vi "From String Array.vi"(8 "error in (no error)":errorcluster, 9 "String Array":string[](array[string]), 11 "Parallel Step Config in":refnum<class "Parallel Step Config.lvclass">) -> (0 "error out":errorcluster, 1 "Elements Left":string[](array[string]), 3 "Parallel Step Config out":refnum<class "Parallel Step Config.lvclass">)   [LabVIEW 2015, in "Parallel Step Config.lvclass"]
uses:
  Parallel Step Config.lvclass
  classes/Step/Config/Step Config.lvclass
panel:
  out "Elements Left 2":string[][](array[string])
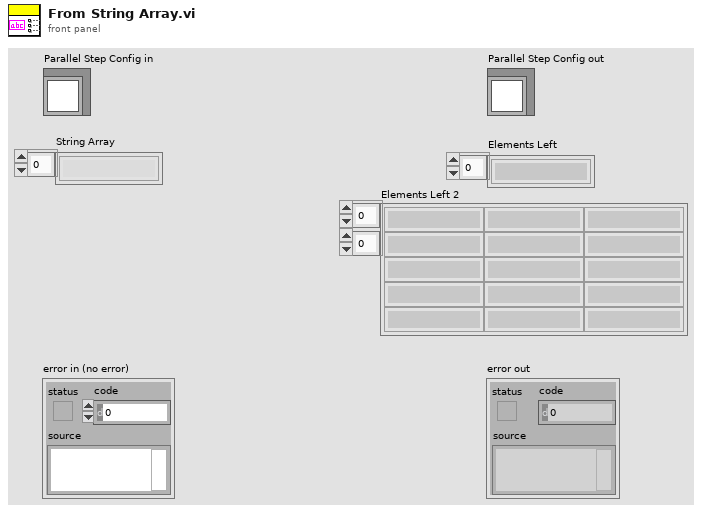
[diagram p1: front panel]
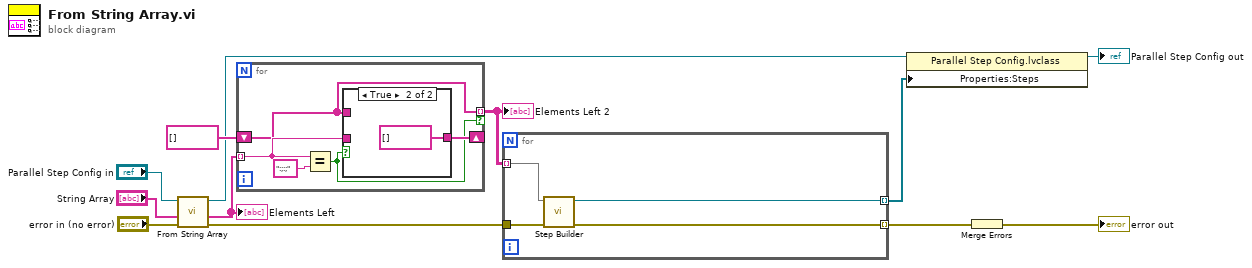
[diagram p0: block diagram]
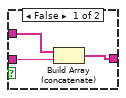
[diagram p2: hidden frame]
diagram:
  n1 = call-parent "From String Array.vi"("error in (no error)"="error in (no error)", "String Array"="String Array", "Step Config in"="Parallel Step Config in") -> ("error out"=w6:errorcluster, "Elements Left 2"=w9:string[], "Step Config out"=w3:refnum<class "Parallel Step Config.lvclass">)  [unwired: 6 in]
  "Elements Left" <- w9
  n2 = for {
    tunnel: w9 -> [w15] mode=indexing
    shift-right: [w16] -> _
    shift-left: string[] [] ("Elements Left 2") -> [w14]
    tunnel: [w14] -> w7 mode=indexing if=w13
    n3 = Equal?(x=w15, y=":;:;") -> (x = y?=w13:bool)
    n4 = case shown="True" w13 {
      tunnel: w14 -> [w20 _]
      tunnel: [w19 string[] []] -> w16
      tunnel: w15 -> [w18 _]
      frame False {
        n5 = Build Array (concatenate)(w20, w18) -> (w19:string[])
      }
      frame True {
      }
    }
  }
  "Elements Left 2" <- w7
  n6 = for {
    tunnel: w7 -> [w25] mode=indexing
    tunnel: w6 -> [w23]
    tunnel: [w22] -> w5 mode=indexing
    tunnel: [w24] -> w1 mode=indexing
    n7 = call "Step Builder.vi"("error in (no error)"=w23, "Standard Sequence"=w25) -> ("error out"=w22:errorcluster, "Step Config out"=w24:refnum<class "Step Config.lvclass">)  [unwired: 8 in]
  }
  n8 = property class="Parallel Step Config.lvclass"(reference=w3, "Properties:Steps"=w1) -> (reference out=→"Parallel Step Config out":refnum<class "Parallel Step Config.lvclass">)  [unwired: 1 in, 1 out]
  n9 = Merge Errors(w5) -> (→"error out":errorcluster)
